vi "Pre Launch Init.vi"(11 "SPIController in":refnum<class "SPIController.lvclass">) -> (0 "error out":errorcluster, 3 "SPIController out":refnum<class "SPIController.lvclass">)   [LabVIEW 2023, in "SPIController.lvlib" / "SPIController.lvclass"]
doc: "(<B>Filename</B>: Actor Framework.lvlib:Actor.lvclass:Pre Launch Init.vi)\n\nDefines behavior that occurs after the Launch Nested Actor method is invoked but before the actor's Actor Core method begins running.\n\nBy default, this method does nothing. A descendant class may override it to define behavior."
uses:
  SPIController.lvclass
  TranslationStage_UI/Arduino_Stepper_UI/Scan_Data_For_Controller.ctl
  SPIController.lvclass/SPIController.ctl
  <vilib>/ActorFramework/Actor/Actor.lvclass
  typedefs/typedefs.lvlib
panel:
  in  "Scan Data":T1
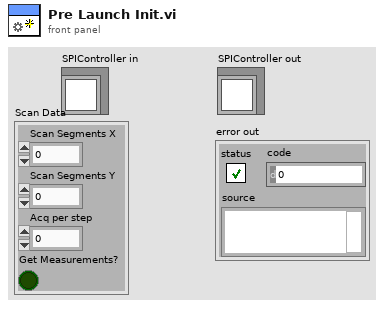
[diagram p1: front panel]
types:
  T1 = typedef "typedefs.lvlib/Scan_Data_For_Controller.ctl" = cluster{"Scan Segments X":u32, "Scan Segments Y":u32, "Acq per step":u8, "Get Measurements?":bool}
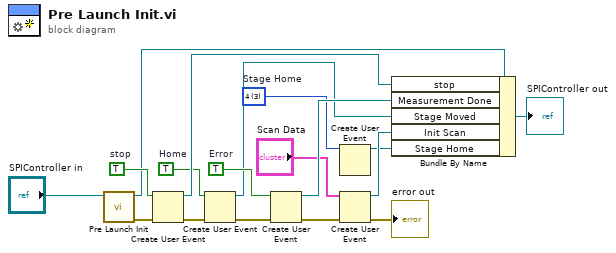
[diagram p0: block diagram]
diagram:
  w3 = u16 3 items=["1", "2", "3", "4"]  # Stage Home
  w7 = TRUE  # Home
  w13 = TRUE  # Error
  w18 = TRUE  # stop
  n1 = call-parent "Pre Launch Init.vi"("Actor in"="SPIController in") -> ("error out"=w10:errorcluster, "Actor out"=w15:refnum<class "SPIController.lvclass">)  [unwired: 9 in]
  n2 = Create User Event(user event datatype=w18, error in=w10) -> (user event=w17:refnum<user-event>, error out=w8:errorcluster)
  n3 = Create User Event(user event datatype=w7, error in=w8) -> (user event=w11:refnum<user-event>, error out=w9:errorcluster)
  n4 = Create User Event(user event datatype=w13, error in=w9) -> (user event=w12:refnum<user-event>, error out=w5:errorcluster)
  n5 = Create User Event(user event datatype=w3) -> (user event=w2:refnum<user-event>)  [unwired: 1 in, 1 out]
  n6 = Create User Event(user event datatype="Scan Data", error in=w5) -> (user event=w6:refnum<user-event>, error out=→"error out":errorcluster)
  n7 = Bundle By Name(cluster=w15, "stop"=w17, "Measurement Done"=w12, "Stage Moved"=w11, "Init Scan"=w6, "Stage Home"=w2) -> (→"SPIController out":refnum<class "SPIController.lvclass">)
